vi "process.vi"(8 "error in (no error)":errorcluster, 11 "DL090216Display in":refnum<class "DisplayDL090216.lvclass">) -> (0 "error out":errorcluster, 2 "finished?":bool, 3 "DL090216Display out":refnum<class "DisplayDL090216.lvclass">)   [LabVIEW 2010, in "DisplayDL090216.lvclass"]
uses:
  DisplayDL090216.lvclass
  DisplayDL090216.lvclass/DisplayDL090216.ctl
  common/classes/Image/Image/Image.lvclass
  ImageProcessor/ImageProcessorDL090216RangeOffset/ImageProcessorDL090216RangeOffset/ImageProcessorDL090216RangeOffset.lvclass
  common/classes/ErrorController/ErrorController/class_data.vi
  common/classes/ErrorController/ErrorController/ErrorController.lvclass
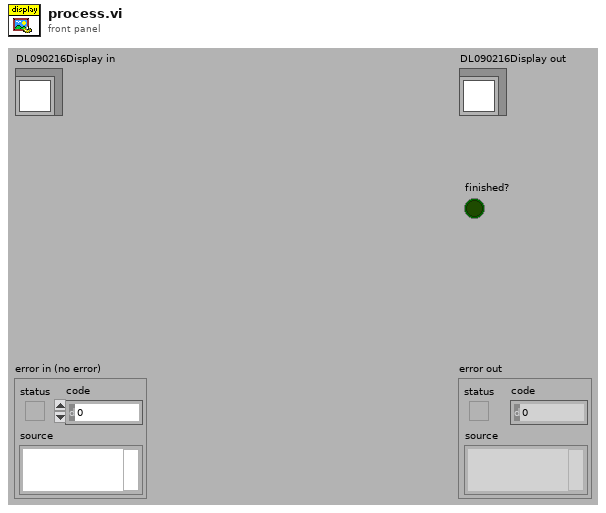
[diagram p1: front panel]
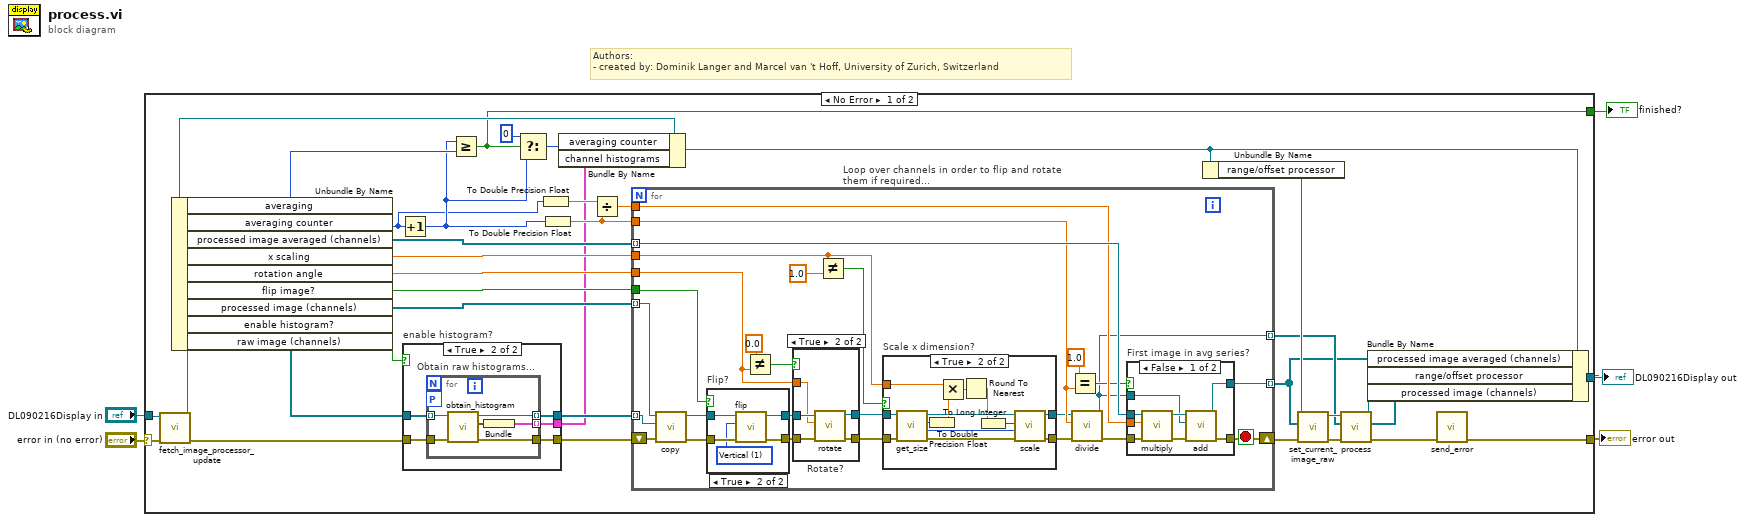
[diagram p0: block diagram]
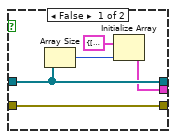
[diagram p2: hidden frame]
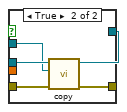
[diagram p3: hidden frame]
diagram:
  # "Authors: \n- created by: Dominik Langer and Marcel van 't Hoff, University of Zurich, Switzerland"
  n1 = case shown="No Error" "error in (no error)" {
    selector: "error in (no error)" -> [w40 w127]
    tunnel: [w35 w127] -> w4
    tunnel: [w7 w126] -> w2
    tunnel: "DL090216Display in" -> [w39 w126]
    tunnel: [w6 _] -> w1
    frame No Error {
      n2 = call-dynamic "fetch_image_processor_update.vi"("error in (no error)"=w40, "DL090216Display in"=w39) -> ("error out"=w36:errorcluster, "DL090216Display out"=w10:refnum<class "DisplayDL090216.lvclass">)  [unwired: 8 out]
      n3 = Unbundle By Name(w10) -> ("averaging"=w27:i32, "averaging counter"=w23:i32, "processed image averaged (channels)"=w31:refnum<class "Image.lvclass">[], "x scaling"=w34:dbl, "rotation angle"=w37:dbl[unit], "flip image?"=w38:bool, "processed image (channels)"=w21:refnum<class "Image.lvclass">[], "enable histogram?"=w32:bool, "raw image (channels)"=w33:refnum<class "Image.lvclass">[])
      n4 = Increment(x=w23) -> (x+1=w24:i32)
      n5 = case "enable histogram?" shown="True" w32 {
        tunnel: w33 -> [w44 w50]
        tunnel: w36 -> [w45 w49]
        tunnel: [w45 w48] -> w22
        tunnel: [w44 w47] -> w20
        tunnel: [w41 w46] -> w12
        frame False {
          n6 = Array Size(array=w44) -> (size(s)=w42:i32)
          n7 = Initialize Array(cluster{"histogram out":cluster{i32, u32}[]} {"histogram out"=[{0, 0}]} ("Cluster"), w42) -> (w41:cluster{"histogram out":cluster{i32, u32}[]}[])
        }
        frame True {
          n8 = for "Obtain raw histograms..." {
            tunnel: w50 -> [w54] mode=indexing
            tunnel: [w52] -> w46 mode=indexing
            tunnel: [w53] -> w47 mode=indexing
            workers-P: _ -> [_]
            tunnel: w49 -> [w56]
            tunnel: [w55] -> w48
            n9 = call "obtain_histogram.vi"("error in (no error)"=w56, "Image in"=w54) -> ("error out"=w55:errorcluster, "histogram out"=w51:cluster{i32, u32}[], "Image out"=w53:refnum<class "Image.lvclass">)  [unwired: 7 in]
            n10 = Bundle("histogram out"=w51) -> (w52:cluster{"histogram out":cluster{i32, u32}[]})  [unwired: 1 in]
          }
        }
      }
      n11 = Greater Or Equal?(x=w24, y=w27) -> (x >= y?=w6:bool)
      n12 = Select(t=0, s=w6, f=w24) -> (s? t:f=w26:i32)
      n13 = To Double Precision Float(number=w23) -> (double precision float=w30:dbl)
      n14 = To Double Precision Float(number=w24) -> (double precision float=w29:dbl)
      n15 = Bundle By Name(cluster=w10, "averaging counter"=w26, "channel histograms"=w12) -> (w9:refnum<class "DisplayDL090216.lvclass">)
      n16 = Divide(x=w30, y=w29) -> (x/y=w28:dbl)
      n17 = for "Loop over channels in order to flip and rotate them if required..." {
        tunnel: w38 -> [w83]
        tunnel: [w63] -> w11 mode=indexing
        tunnel: w37 -> [w78]
        tunnel: w34 -> [w75]
        shift-right: [w71] -> w17
        shift-left: w22 -> [w60]
        tunnel: w29 -> [w67]
        tunnel: w31 -> [w69] mode=indexing
        tunnel: w28 -> [w68]
        tunnel: w20 -> [w62] mode=indexing
        tunnel: w21 -> [w61] mode=indexing
        tunnel: [w57] -> w14 mode=indexing
        stop <- w71 stop-if-true
        n18 = call "copy.vi"("error in (no error)"=w60, "image to copy (source)"=w62, "Image in (target)"=w61) -> ("error out"=w59:errorcluster, "Image out"=w58:refnum<class "Image.lvclass">)  [unwired: 7 in]
        n19 = case "Flip?" shown="True" w83 {
          tunnel: w59 -> [w120 w125]
          tunnel: [w120 w124] -> w82
          tunnel: [w119 w123] -> w81
          tunnel: w58 -> [w119 w121]
          frame False {
          }
          frame True {
            w122 = u32 1 items=["Horizontal", "Vertical", "Central", "1st Diagonal", "2nd Diagonal"] ("Type of Symmetry")
            n20 = call "flip.vi"("error in (no error)"=w125, "Type of Symmetry"=w122, "Image in"=w121) -> ("error out"=w124:errorcluster, "Image out"=w123:refnum<class "Image.lvclass">)  [unwired: 7 out]
          }
        }
        n21 = Not Equal?(x=dbl[unit] 0.0 ("y"), y=w78) -> (x != y?=w80:bool)
        n22 = case "Rotate?" shown="True" w80 {
          tunnel: w82 -> [w112 w118]
          tunnel: w81 -> [w113 w117]
          tunnel: [w113 w116] -> w77
          tunnel: [w112 w115] -> w76
          tunnel: w78 -> [_ w114]
          frame False {
          }
          frame True {
            n23 = call "rotate.vi"("error in (no error)"=w118, "angle"=w114, "Image in"=w117) -> ("error out"=w115:errorcluster, "Image out"=w116:refnum<class "Image.lvclass">)  [unwired: 7 out]
          }
        }
        n24 = Not Equal?(x=w75, y=1.0) -> (x != y?=w73:bool)
        n25 = case "Scale x dimension?" shown="True" w73 {
          tunnel: w77 -> [w98 w111]
          tunnel: w76 -> [w97 w110]
          tunnel: [w97 w108] -> w72
          tunnel: [w98 w106] -> w64
          tunnel: w75 -> [_ w104]
          frame False {
          }
          frame True {
            n26 = call-dynamic "get_size.vi"("error in (no error)"=w110, "Image in"=w111) -> ("error out"=w109:errorcluster, "y resolution"=w105:i32, "x resolution"=w103:i32, "Image out"=w107:refnum<class "Image.lvclass">)  [unwired: 2 in, 4 out]
            n27 = To Double Precision Float(number=w103) -> (double precision float=w102:dbl)
            n28 = Multiply(x=w104, y=w102) -> (x*y=w101:dbl)
            n29 = Round To Nearest(number=w101) -> (nearest integer value=w100:dbl)
            n30 = To Long Integer(number=w100) -> (32bit integer=w99:i32)
            n31 = call-dynamic "scale.vi"("error in (no error)"=w109, "y"=w105, "x"=w99, "Image in"=w107) -> ("error out"=w108:errorcluster, "Image out"=w106:refnum<class "Image.lvclass">)  [unwired: 6 in]
          }
        }
        n32 = Equal?(x=1.0, y=w67) -> (x = y?=w65:bool)
        n33 = call-dynamic "divide.vi"("error in (no error)"=w72, "divisor"=w67, "Image in"=w64) -> ("error out"=w70:errorcluster, "Image out"=w57:refnum<class "Image.lvclass">)  [unwired: 7 in]
        n34 = case "First image in avg series?" shown="False" w65 {
          tunnel: [w86 w93] -> w63
          tunnel: [w84 w95] -> w71
          tunnel: w70 -> [w91 w96]
          tunnel: w69 -> [w89 w94]
          tunnel: w57 -> [w85 w92]
          tunnel: w68 -> [w87 _]
          frame False {
            n35 = call-dynamic "multiply.vi"("error in (no error)"=w91, "factor"=w87, "Image in"=w89) -> ("error out"=w90:errorcluster, "Image out"=w88:refnum<class "Image.lvclass">)  [unwired: 7 in]
            n36 = call-dynamic "add.vi"("error in (no error)"=w90, "addend"=w85, "Image in"=w88) -> ("error out"=w84:errorcluster, "Image out"=w86:refnum<class "Image.lvclass">)  [unwired: 7 in]
          }
          frame True {
            n37 = call "copy.vi"("error in (no error)"=w96, "image to copy (source)"=w92, "Image in (target)"=w94) -> ("error out"=w95:errorcluster, "Image out"=w93:refnum<class "Image.lvclass">)  [unwired: 7 in]
          }
        }
      }
      n38 = Unbundle By Name(w9) -> ("range/offset processor"=w15:refnum<class "ImageProcessorDL090216RangeOffset.lvclass">)
      n39 = call-dynamic "set_current_image_raw.vi"("error in (no error)"=w17, "current image raw (channels)"=w11, "GenericImageProcessor.lvclass in"=w15) -> ("error out"=w18:errorcluster, "GenericImageProcessor.lvclass out"=w19:refnum<class "ImageProcessorDL090216RangeOffset.lvclass">)  [unwired: 7 out]
      n40 = call-dynamic "process.vi"("error in (no error)"=w18, "destination image in (channels)"=w14, "DL090216RangeOffsetImageProcessor in"=w19) -> ("error out"=w16:errorcluster, "destination image out (channels)"=w8:refnum<class "Image.lvclass">[], "DL090216RangeOffsetImageProcessor out"=w13:refnum<class "ImageProcessorDL090216RangeOffset.lvclass">)  [unwired: 6 out]
      n41 = Bundle By Name(cluster=w9, "processed image averaged (channels)"=w11, "range/offset processor"=w13, "processed image (channels)"=w8) -> (w7:refnum<class "DisplayDL090216.lvclass">)
      n42 = call "send_error.vi"("error in (no error)"=w16) -> ("error out"=w35:errorcluster)  [unwired: 10 in]
    }
    frame Error {
    }
  }
  "error out" <- w4
  "DL090216Display out" <- w2
  "finished?" <- w1
